vi "Get 2-Byte Integer.vi"(11 "Bytes in":u8[](array[numeric])) -> (1 "2-Byte Integer":u64, 3 "Bytes out":u8[](array[numeric]))   [LabVIEW 2014, in "hse-db.lvlib" / "MySQL (TCP).lvlib"]
uses:
  MySQL (TCP).lvlib
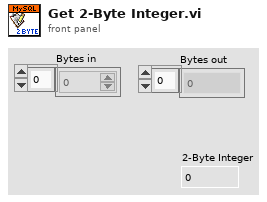
[diagram p1: front panel]
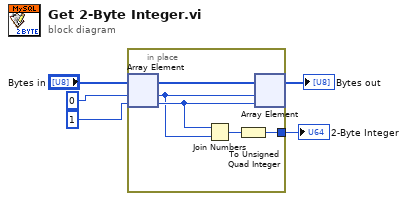
[diagram p0: block diagram]
diagram:
  n1 = in-place {
    in-place-border: [w8] -> w4
    n2 = in-place-array #1("Bytes in", 0, 1) -> (w5:u8, w6:u8)
    n3 = Join Numbers(hi=w6, lo=w5) -> ((hi.lo)=w7:u16)
    n4 = To Unsigned Quad Integer(1:w7) -> (0:w8:u64)
    n5 = in-place-array #1(w5, w6) -> ()  [unwired: 3 out]
  }
  "2-Byte Integer" <- w4
  "Bytes out" <- "Bytes in"
